vi "Read IncDec Visible.vi"(9 "Digital in":refnum<class "Digital.lvclass">) -> (3 "Digital out":refnum<class "Digital.lvclass">, 4 "IncDec Visible":bool)   [LabVIEW 2014, in "Digital.lvclass"]
uses:
  Digital.lvclass
  Digital.lvclass/Digital.ctl
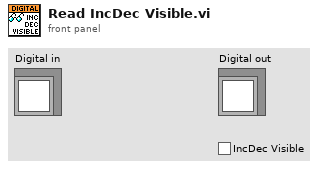
[diagram p1: front panel]
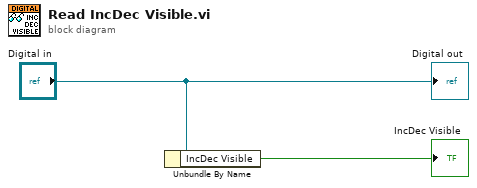
[diagram p0: block diagram]
diagram:
  n1 = Unbundle By Name("Digital in") -> ("IncDec Visible"=→"IncDec Visible":bool)
  "Digital out" <- "Digital in"
